vi "Read Result Channel.vi"(8 "error in (no error)":errorcluster, 11 "String Compare Config in":refnum<class "String Compare Config.lvclass">) -> (0 "error out":errorcluster, 2 "channel":refnum<class "TBM channel.lvclass">, 3 "String Compare Config out":refnum<class "String Compare Config.lvclass">)   [LabVIEW 2015, in "String Compare Config.lvclass"]
uses:
  String Compare Config.lvclass
  <vilib>/NI/Tag Bus Module Framework/channel/TBM channel.lvclass
  String Compare Config.lvclass/String Compare Config.ctl
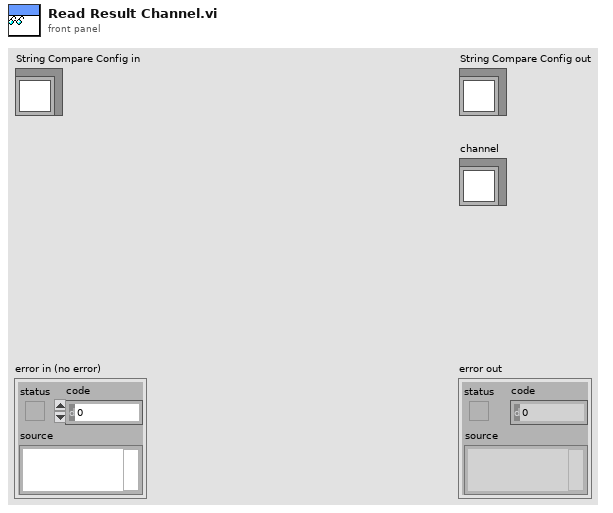
[diagram p1: front panel]
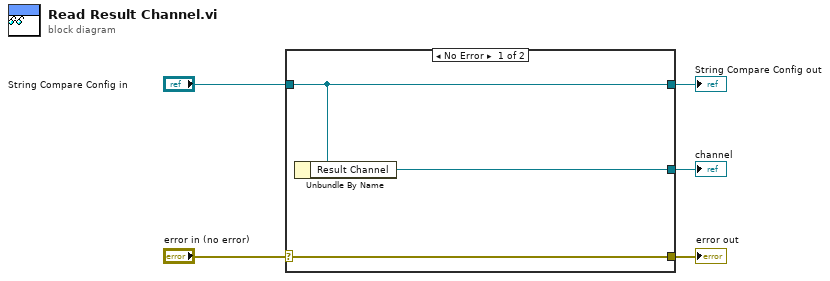
[diagram p0: block diagram]
diagram:
  n1 = case shown="No Error" "error in (no error)" {
    selector: "error in (no error)" -> [w8 w9]
    tunnel: [w8 w9] -> w4
    tunnel: [w7 w10] -> w2
    tunnel: "String Compare Config in" -> [w7 w10]
    tunnel: [w6 _] -> w1
    frame No Error {
      n2 = Unbundle By Name(w7) -> ("Result Channel"=w6:refnum<class "TBM channel.lvclass">)
    }
    frame Error {
    }
  }
  "error out" <- w4
  "String Compare Config out" <- w2
  "channel" <- w1
